vi "Actor Core.vi"(8 "error in":errorcluster, 11 "Nested in":refnum<class "MSS Host Actor.lvclass">) -> (0 "error out":errorcluster, 3 "Actor out":refnum<class "Actor.lvclass">)   [LabVIEW 2023, in "MSS Host Actor.lvlib" / "MSS Host Actor.lvclass"]
doc: "(<B>Filename</B>: Actor Framework.lvlib:Actor.lvclass:Actor Core.vi)\n\nReceives messages to the actor, reacts to them, and initiates any error handling that may shut the actor down.\n\nDescendant classes may override this VI to append parallel tasks for the actor to complete while it handles messages. Overrides use the Call Parent Method node."
uses:
  MSS Host Actor.lvclass
  <vilib>/ActorFramework/Actor/Actor.lvclass
  <vilib>/ni/Actors/Network Endpoint Actors/Notifying Nested Endpoint/Notifying Nested Endpoint.lvclass
  <vilib>/ActorFramework/Actor/Actor.lvclass/Actor.ctl
  <vilib>/ActorFramework/Message Enqueuer/Message Enqueuer.lvclass/Message Enqueuer.ctl
  MSS Host Actor.lvclass/MSS Host Actor.ctl
  <vilib>/ni/Actors/Network Endpoint Actors/Network Endpoint/Network Endpoint/Network Endpoint.lvclass/Network Endpoint.ctl
  MSS Host Actor Messages/Read and Send Configuration Msg/Read and Send Configuration Msg.lvclass/Read and Send Configuration Msg.ctl
  <vilib>/ActorFramework/Message Enqueuer/Init from Existing Queue.vi
  <vilib>/ActorFramework/Message Enqueuer/Enqueue.vi
  <vilib>/ActorFramework/Stop Msg/Stop Msg.lvclass
  MSS Host Actor Messages/Read and Send Configuration Msg/Read and Send Configuration Msg.lvclass
  <vilib>/Utility/LVClass/Get LV Class Name.vi
  <resource>/AFDebug/Generate Trace for Message.vi
  <vilib>/ActorFramework/Message Priority Queue/Priority Enqueue.vi
  <userlib>/_OpenG.lib/file/file.llb/Valid Path - Traditional__ogtk.vi
  <userlib>/_OpenG.lib/file/file.llb/Valid Path - Array__ogtk.vi
  <vilib>/ActorFramework/Message Enqueuer/Message Enqueuer.lvclass
  AF Helpers/My Actor/My Actor/My Actor.lvclass
  <userlib>/_OpenG.lib/file/file.llb/openg_file.lvlib
  <vilib>/ni/Actors/Network Endpoint Actors/Network Endpoint/Network Endpoint/Network Endpoint.lvclass
panel:
  out "Connected":bool
  in  "Excitation":T1
  in  "Start Button":bool
  in  "Intrs":T2
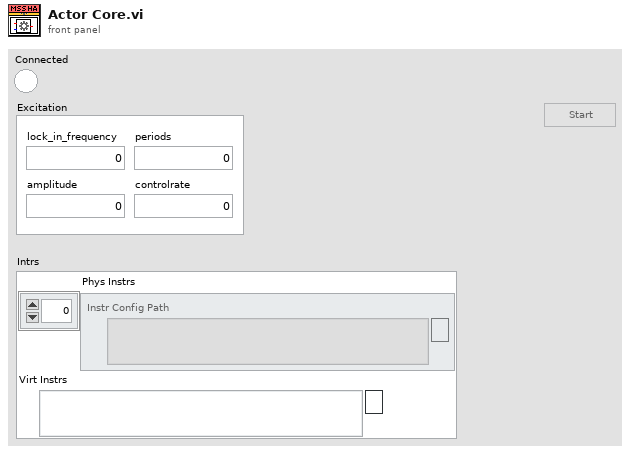
[diagram p1: front panel]
types:
  T1 = cluster{"lock_in_frequency":dbl, "amplitude":dbl, "periods":dbl, "controlrate":dbl}
  T2 = cluster{"Phys Instrs":path[], "Virt Instrs":path}
  T3 = cluster{"Stop":refnum<user-event>, "Connected":refnum<user-event>}
  T4 = enum8{"Enabled", "Disabled", "Disabled and Grayed Out"}
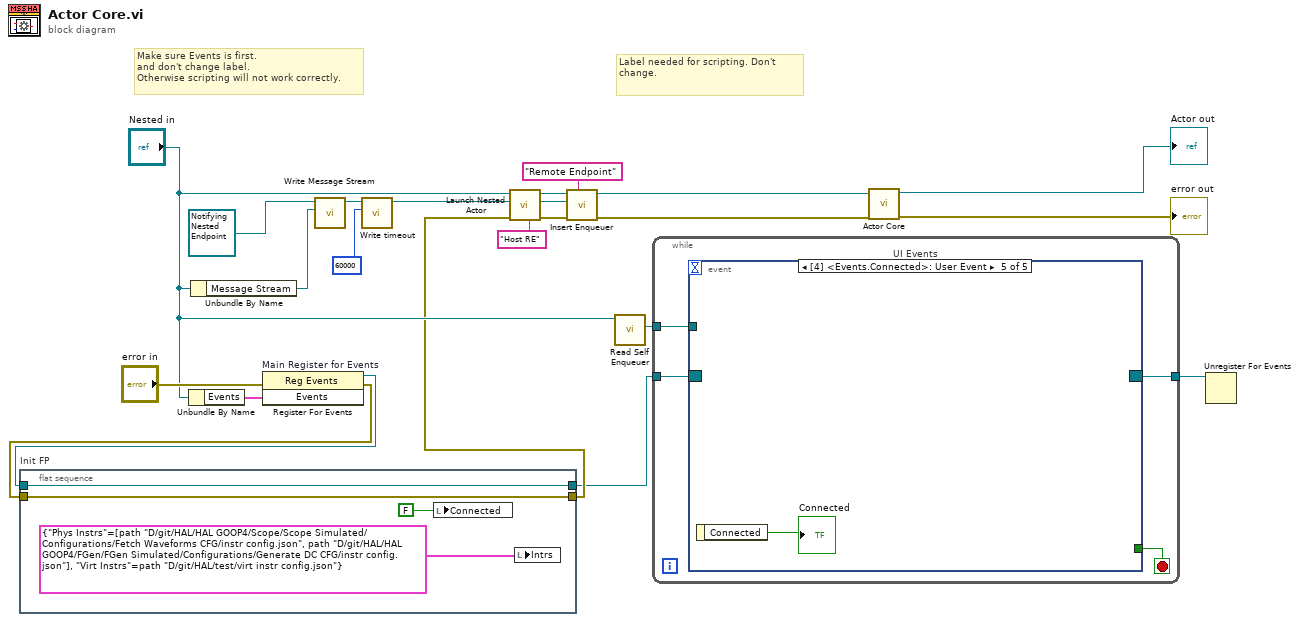
[diagram p0: block diagram]
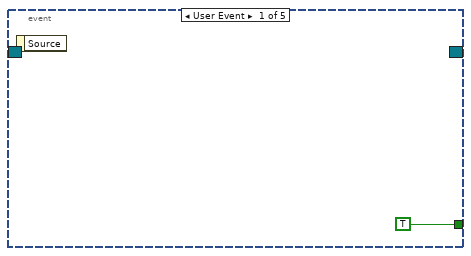
[diagram p2: hidden frame]
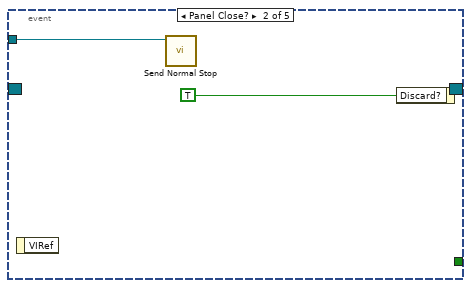
[diagram p3: hidden frame]
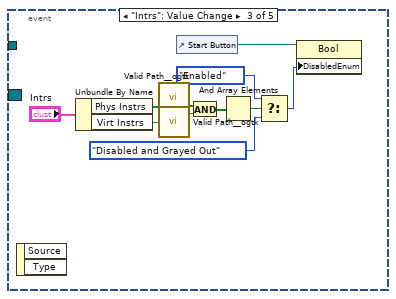
[diagram p4: hidden frame]
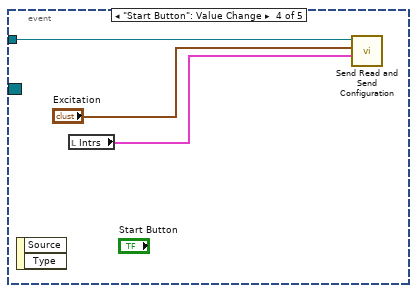
[diagram p5: hidden frame]
diagram:
  # "Label needed for scripting. Don't change."
  # "Make sure Events is first.\nand don't change label.\nOtherwise scripting will not work correctly."
  n1 = flat-sequence "Init FP" {
    tunnel: w5 -> [w25]
    tunnel: [w25] -> w4
    tunnel: w3 -> [w24]
    tunnel: [w24] -> w2
    frame #0 {
      n2 = local write "Connected"(FALSE ("Connected")) -> ()
      n3 = local write "Intrs"(T2 {"Phys Instrs"=[path "D:/git/HAL/HAL GOOP4/Scope/Scope Simulated/Configurations/Fetch Waveforms CFG/instr config.json", path "D:/git/HAL/HAL GOOP4/FGen/FGen Simulated/Configurations/Generate DC CFG/instr config.json"], "Virt Instrs"=path "D:/git/HAL/test/virt instr config.json"} ("Intrs")) -> ()
    }
  }
  n4 = Unbundle By Name("Nested in") -> ("Events"=w21:T3)
  n5 = Unbundle By Name("Nested in") -> ("Message Stream"=w15:refnum<class "Message Stream.lvclass">)
  n6 = register-events "Main Register for Events"(error in="error in", w21) -> (reference out=w3:refnum<event-registration>, error out=w5:errorcluster)  [unwired: 1 in]
  n7 = call <vilib>:"Write Message Stream.vi"("Message Stream"=w15, "Network Endpoint in"=refnum<class "Notifying Nested Endpoint.lvclass"> refnum ("Notifying Nested Endpoint.lvclass")) -> ("Network Endpoint out"=w17:refnum<class "Notifying Nested Endpoint.lvclass">)  [unwired: 9 in]
  n8 = call <vilib>:"Write timeout.vi"("timeout"=60000, "Network Endpoint in"=w17) -> ("Network Endpoint out"=w12:refnum<class "Notifying Nested Endpoint.lvclass">)  [unwired: 9 in]
  n9 = call <vilib>:"Launch Nested Actor.vi"("Debug Alias"="Host RE", "error in (no error)"=w4, "Nested Actor"=w12, "Caller Actor in"="Nested in") -> ("error out"=w11:errorcluster, "Nested Actor's Enqueuer"=w7:refnum<class "Message Enqueuer.lvclass">, "Caller Actor out"=w9:refnum<class "MSS Host Actor.lvclass">)  [unwired: 5 in]
  n10 = call-dynamic "Insert Enqueuer.vi"("Enqueuer Ident"="Remote Endpoint", "error in (no error)"=w11, "Nested Actor's Enqueuer"=w7, "My Actor in"=w9) -> ("error out"=w10:errorcluster, "My Actor out"=w8:refnum<class "MSS Host Actor.lvclass">)  [unwired: 6 in]
  n11 = call <vilib>:"Read Self Enqueuer.vi"("Actor"="Nested in") -> ("Self Enqueuer"=w19:refnum<class "Message Enqueuer.lvclass">)  [unwired: 10 in]
  n12 = while {
    tunnel: w2 -> [w31]
    tunnel: [w29] -> w20
    tunnel: w19 -> [w28]
    stop <- w30 stop-if-true
    n13 = event "UI Events" shown="[4] <Events.Connected>: User Event" {
      selector: w31 -> [_ _ _ _ _]
      dyn-events: [_ _ _ _ _] -> w29
      timeout: _ -> [_ _ _ _ _]
      tunnel: [TRUE _ _ _ _] -> w30
      tunnel: w28 -> [_ w33 _ w48 _]
      event User Event {
        n14 = event-data() -> ()  [unwired: 1 in, 1 out]
      }
      event Panel Close? {
        n15 = event-data() -> ()  [unwired: 1 in, 1 out]
        n16 = call <vilib>:"Send Normal Stop.vi"("Message Enqueuer"=w33) -> ()  [unwired: 10 in, 1 out]
        n17 = event-data("Discard?"=TRUE) -> ()  [unwired: 1 in, 1 out]
      }
      event "Intrs": Value Change {
        n18 = event-data() -> ()  [unwired: 1 in, 2 out]
        n19 = Unbundle By Name("Intrs") -> ("Phys Instrs"=w44:path[], "Virt Instrs"=w45:path)
        n20 = call-poly <userlib>:"Valid Path__ogtk.vi"("array of paths"=w44) -> ("valid"=w42:bool[])
        n21 = call-poly <userlib>:"Valid Path__ogtk.vi"("path"=w45) -> ("valid"=w43:bool)
        n22 = control-ref of="Start Button"() -> (w39:refnum<vi>)
        n23 = And(x=w42, y=w43) -> (x .and. y?=w41:bool[])
        n24 = And Array Elements(Boolean array=w41) -> (logical AND=w38:bool)
        n25 = Select(t=T4."Enabled" ("Disabled"), s=w38, f=T4."Disabled and Grayed Out" ("Disabled")) -> (s? t:f=w36:T4)
        n26 = property class="Bool"(reference=w39, "DisabledEnum"=w36) -> ()  [unwired: 1 in, 2 out]
      }
      event "Start Button": Value Change {
        n27 = event-data() -> ()  [unwired: 1 in, 2 out]
        n28 = local read "Intrs"() -> (w46:T2)
        n29 = call "Send Read and Send Configuration.vi"("Intrs"=w46, "Excitation"="Excitation", "Message Enqueuer"=w48) -> ()  [unwired: 7 in, 2 out]
      }
      event User Event {
        n30 = event-data() -> ("Connected"=→"Connected":bool)  [unwired: 1 in]
      }
    }
  }
  n31 = call-parent "Actor Core.vi"("error in"=w10, "Actor in"=w8) -> ("error out"=→"error out":errorcluster, "Actor out"=→"Actor out":refnum<class "Actor.lvclass">)  [unwired: 8 in]
  n32 = Unregister For Events(event registration refnum=w20) -> ()  [unwired: 1 in, 1 out]
